vi "quest-about.vi"() -> ()   [LabVIEW 2019]
panel:
  in  "stop":bool
  # "About"
  # "La integridad de este programa de labview ha sido desarrollado por Francisco Javier Encabo Fernández. Dicho gilipollas es un\nputo FPII que por más que se esfuerce en su trabajo siempre será un puto FPII. Y cuál es la solución que le ofrecen los \"jefes\" a este moñas... SACATE UN PLAZA LIBRE DE FUNCIONARIO, y como se siente el último puto mono después de tan buena solución, pues te lo digo:\nDesesperado.\nDesilusionado.\nDesanimado.\nDesmotivado.\nDesamparado.\nDesapegado.\nEngañado.\nDesgraciado.\nDespreciado.\nDesafortunado.\nDescartado.\nDesdichado.\nNinguneado.\n...\n...\netc..\n\nY así podría seguir con más vocablos.\nAsí que tenemos varias opciones, la primera sigo haciendo las cosas con esfuerzo, cuidando cada detalle, mimando el código y poniendo todo mi cariño.... de esta forma mis posibilidades de promoción y de reconocimiento  seguirán siendo las mismas.. NINGUNA.\nLa segunda solución es pasar de todo, hacer los programas deprisa y corriendo, no comentar  ningún código, que me de lo mismo que funcione perfectamente y en definitiva no esforzarme por hacer mi trabajo limpiamente (aunque así es como trabajan aquí), de esta forma mis posibilidades de promoción y ascenso son las mismas en la anterior ósea NINGUNA, pero al menos no me sentiré como la mierda que ahora me siento por hacer las cosas bien sin reconocimiento.\nEn definitiva al que mantenga este codigo que sepa que esta mal echo, no por que no supiera hacerlo mucho mejor (que si lo se hacer), sino por que no me da la gana hacerlo mejor. Y todo por que el ciemat me otorga un nivel que no corresponde con el trabajo que desempeño.\n\nFirmado el mas gilipollas y ultimo mono del CIEMAT."
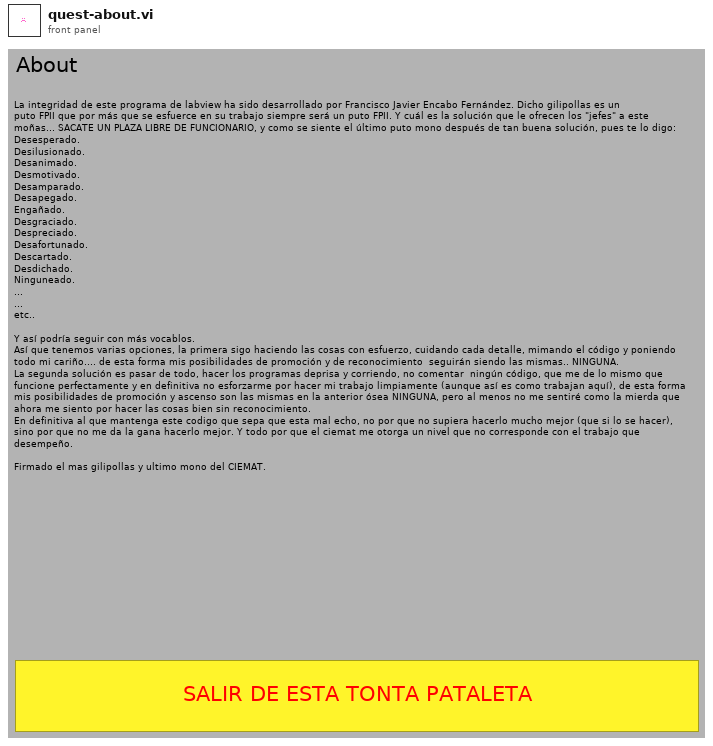
[diagram p1: front panel]
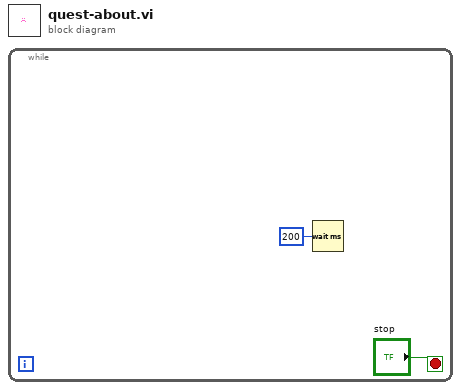
[diagram p0: block diagram]
diagram:
  n1 = while {
    stop <- "stop" stop-if-true
    n2 = Wait (ms)(milliseconds to wait=u32 200) -> ()  [unwired: 1 out]
  }
